vi "BuildInterfData.vi"(8 "error in":errorcluster caption="entrée d'erreur (pas d'erreur)", 10 "IndCourbe":i64, 11 "Experiment.lvclass In":refnum<class "Experiment.lvclass">) -> (0 "error out":errorcluster caption="sortie d'erreur", 1 "NomDon":string[](array[string])=["RTêta;", "X&Y;"], 2 "Scan list":string[](array[string]), 3 "ArrDev":bool[](array[boolean]), 4 "VarPar list":string[](array[string]), 5 "VarParams":string[][](array[string]), 6 "ScanInstIndexOut":i32[][](array[numeric]))   [LabVIEW 2019, in "Experiment.lvclass"]
uses:
  Experiment.lvclass
  Experiment.lvclass/Experiment.ctl
  DevicesClass/BaseDevice/BaseDevice.lvclass
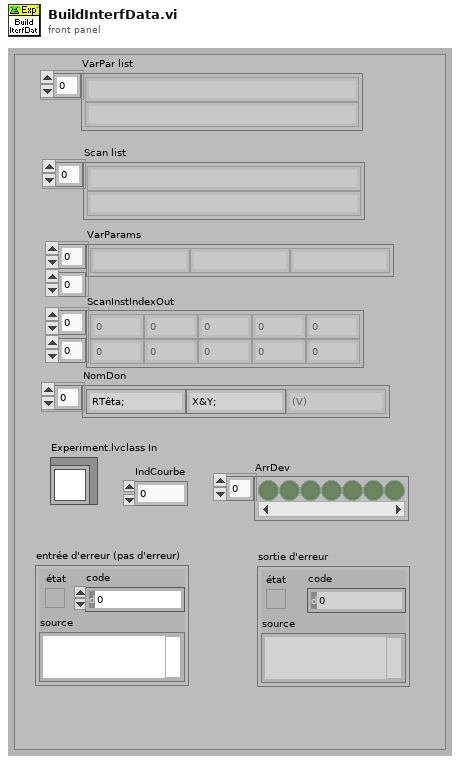
[diagram p1: front panel]
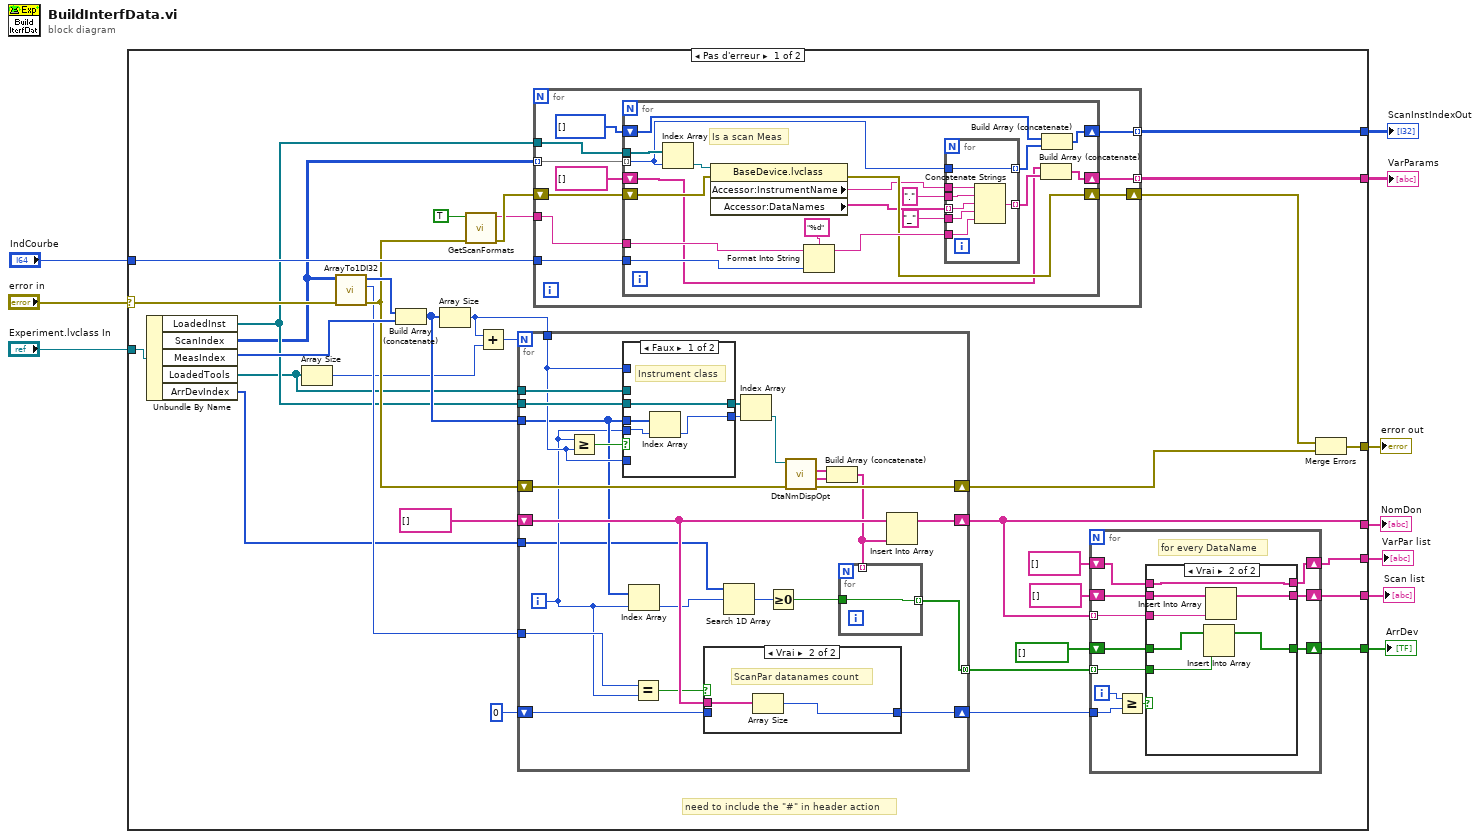
[diagram p0: block diagram]
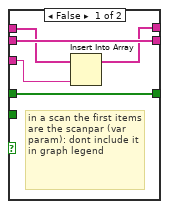
[diagram p2: hidden frame]
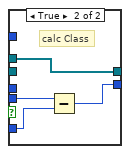
[diagram p3: hidden frame]
diagram:
  n1 = case shown="Pas d'erreur" "error in" {
    selector: "error in" -> [w44 w141]
    tunnel: [w37 w141] -> w9
    tunnel: [w40 _] -> w8
    tunnel: "Experiment.lvclass In" -> [w43 _]
    tunnel: [w39 _] -> w6
    tunnel: "IndCourbe" -> [w38 _]
    tunnel: [w35 _] -> w4
    tunnel: [w16 _] -> w3
    tunnel: [w13 _] -> w2
    tunnel: [w11 _] -> w1
    frame No Error {
      # "need to include the \"#\" in header action"
      n2 = Unbundle By Name(w43) -> ("LoadedInst"=w23:refnum<class "BaseDevice.lvclass">[], "ScanIndex"=w12:i32[][], "MeasIndex"=w42:i32[], "LoadedTools"=w22:refnum<class "BaseDevice.lvclass">[], "ArrDevIndex"=w18:i32[])
      n3 = Array Size(array=w22) -> (size(s)=w21:i32)
      n4 = call <userlib>:"ArrayTo1DI32.vi"("ErrorIn(No Error)"=w44, "tableau"=w12) -> ("sortie d'erreur"=w29:errorcluster, "Size"=w28:i32, "Array Out"=w33:i32[])  [unwired: 7 in]
      n5 = Build Array (concatenate)(w33, w42) -> (w24:i32[])
      n6 = Array Size(array=w24) -> (size(s)=w19:i32)
      n7 = call "GetScanFormats.vi"("ErrorIn(No Error)"=w29, "Scan(T)"=TRUE) -> ("sortie d'erreur"=w31:errorcluster, "Prefixe"=w30:string)  [unwired: 7 in, 1 out]
      n8 = Add(x=w19, y=w21) -> (x+y=w20:i32)
      n9 = for {
        N: w20 -> [_]
        shift-right: [w127] -> w40
        shift-left: string[] [] -> [w126]
        tunnel: w24 -> [w113]
        shift-right: [w125] -> w41
        shift-left: w29 -> [w128]
        tunnel: w28 -> [w124]
        shift-right: [w123] -> w26
        shift-left: 0 -> [w122]
        tunnel: w23 -> [w117]
        tunnel: w22 -> [w115]
        tunnel: w19 -> [w114]
        tunnel: w18 -> [w111]
        tunnel: [w107] -> w17 mode=concatenating
        i -> [w112]
        n10 = Greater Or Equal?(x=w112, y=w114) -> (x >= y?=w116:bool)
        n11 = case shown="Faux" w116 {
          tunnel: w113 -> [w133 _]
          tunnel: [w132 w134] -> w119
          tunnel: [w131 w137] -> w118
          tunnel: w117 -> [w131 _]
          tunnel: w115 -> [_ w137]
          tunnel: w114 -> [_ _]
          tunnel: w112 -> [w130 w136]
          tunnel: w114 -> [_ w135]
          frame False {
            # "Instrument class"
            n12 = Index Array(array=w133, index=w130) -> (element=w132:i32)
          }
          frame True {
            # "calc Class"
            n13 = Subtract(x=w136, y=w135) -> (x-y=w134:i32)
          }
        }
        n14 = Index Array(array=w113, index=w112) -> (element=w110:i32)
        n15 = Equal?(x=w124, y=w112) -> (x = y?=w121:bool)
        n16 = case shown="Vrai" w121 {
          tunnel: w126 -> [_ w140]
          tunnel: [w138 w139] -> w123
          tunnel: w122 -> [w138 _]
          frame False {
          }
          frame True {
            # "ScanPar datanames count"
            n17 = Array Size(array=w140) -> (size(s)=w139:i32)
          }
        }
        n18 = Search 1D Array(1D array=w111, element=w110) -> (index of element=w109:i32)  [unwired: 1 in]
        n19 = Index Array(array=w118, index=w119) -> (element=w120:refnum<class "BaseDevice.lvclass">)
        n20 = Greater Or Equal To 0?(x=w109) -> (x >= 0?=w108:bool)
        n21 = call "DtaNmDispOpt.vi"("error in (no error)"=w128, "BaseDevice en entrée"=w120) -> ("error out"=w125:errorcluster, "ArrDisplayNames"=w104:string[], "DisplayNames"=w106:string[])  [unwired: 6 in, 1 out]
        n22 = Build Array (concatenate)(w106, w104) -> (w105:string[])
        n23 = for {
          tunnel: w108 -> [w129]
          tunnel: [w129] -> w107 mode=indexing
          tunnel: w105 -> [_] mode=indexing
        }
        n24 = Insert Into Array(array=w126, new element=w105) -> (w127:string[])  [unwired: 1 in]
      }
      n25 = for {
        tunnel: w12 -> [w77] mode=indexing
        shift-right: [w72] -> w36
        shift-left: w31 -> [w75]
        tunnel: [w73] -> w39 mode=indexing
        tunnel: w23 -> [w76]
        tunnel: w30 -> [w71]
        tunnel: w38 -> [w70]
        tunnel: [w68] -> w11 mode=indexing
        n26 = for {
          tunnel: w77 -> [w81] mode=indexing
          tunnel: w76 -> [w96]
          shift-right: [w87] -> w72
          shift-left: w75 -> [w88]
          shift-right: [w93] -> w73
          shift-left: string[] [] -> [w82]
          tunnel: w71 -> [w91]
          tunnel: w70 -> [w85]
          shift-right: [w79] -> w68
          shift-left: i32[] [] -> [w78]
          # "Is a scan Meas"
          n27 = Index Array(array=w96, index=w81) -> (element=w86:refnum<class "BaseDevice.lvclass">)
          n28 = property class="BaseDevice.lvclass"(reference=w86, error in=w88) -> (error out=w87:errorcluster, "Accessor:InstrumentName"=w84:string, "Accessor:DataNames"=w83:string[])  [unwired: 1 out]
          n29 = Format Into String(format string="%d" ("chaîne de format"), initial string=w91, w85) -> (resulting string=w89:string)  [unwired: 1 in, 1 out]
          n30 = for {
            tunnel: w83 -> [w103] mode=indexing
            tunnel: "." ("chaîne") -> [w102]
            tunnel: [w101] -> w94 mode=indexing
            tunnel: w84 -> [w100]
            tunnel: "_" ("chaîne") -> [w99]
            tunnel: w89 -> [w98]
            tunnel: w81 -> [w97]
            tunnel: [w97] -> w80 mode=indexing
            n31 = Concatenate Strings(w100, w102, w103, w99, w98) -> (w101:string)
          }
          n32 = Build Array (concatenate)(w82, w94) -> (w93:string[])
          n33 = Build Array (concatenate)(w78, w80) -> (w79:i32[])
        }
      }
      n34 = for {
        tunnel: w40 -> [w53] mode=indexing
        shift-right: [w54] -> w35
        shift-left: string[] [] -> [w55]
        tunnel: w26 -> [w50]
        tunnel: w17 -> [w48] mode=indexing
        shift-right: [w49] -> w16
        shift-left: bool[] [] -> [w47]
        shift-right: [w45] -> w13
        shift-left: string[] [] -> [w46]
        i -> [w51]
        # "for every DataName"
        n35 = Greater Or Equal?(x=w51, y=w50) -> (x >= y?=w52:bool)
        n36 = case shown="Vrai" w52 {
          tunnel: w55 -> [w60 w67]
          tunnel: [w60 w66] -> w54
          tunnel: w53 -> [w57 w65]
          tunnel: [w59 w62] -> w49
          tunnel: w48 -> [_ w63]
          tunnel: w47 -> [w59 w64]
          tunnel: w46 -> [w58 w61]
          tunnel: [w56 w61] -> w45
          frame False {
            # "in a scan the first items are the scanpar (var param): dont include it in graph legend"
            n37 = Insert Into Array(array=w58, new element=w57) -> (w56:string[])  [unwired: 1 in]
          }
          frame True {
            n38 = Insert Into Array(array=w64, new element=w63) -> (w62:bool[])  [unwired: 1 in]
            n39 = Insert Into Array(array=w67, new element=w65) -> (w66:string[])  [unwired: 1 in]
          }
        }
      }
      n40 = Merge Errors(w36, w41) -> (w37:errorcluster)
    }
    frame Error {
    }
  }
  "error out" <- w9
  "NomDon" <- w8
  "VarParams" <- w6
  "Scan list" <- w4
  "ArrDev" <- w3
  "VarPar list" <- w2
  "ScanInstIndexOut" <- w1
